vi "MSScript_SubVI_ArrayIndiceString.vi"(11 "indice string in":string) -> (1 "x:y":i32[](array[numeric]), 2 "Indice string?":bool, 3 "Array indice string out":string)   [LabVIEW 2018, in "MSScript.lvclass"]
uses:
  MSScript.lvclass
  MSScript_Transform_UInt.vi
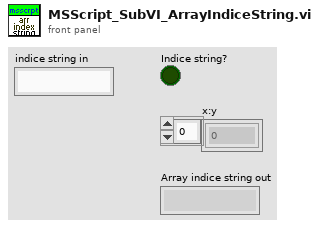
[diagram p1: front panel]
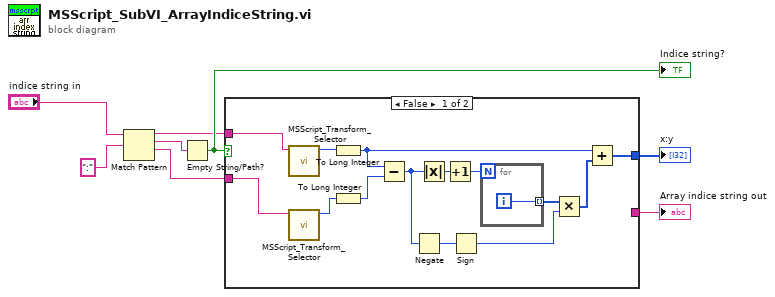
[diagram p0: block diagram]
diagram:
  n1 = Match Pattern(string="indice string in", regular expression=":") -> (before substring=w3:string, match substring=w2:string, after substring=w4:string)  [unwired: 1 in, 1 out]
  n2 = Empty String/Path?(string/path=w2) -> (empty?=w6:bool)
  "Indice string?" <- w6
  n3 = case shown="False" w6 {
    tunnel: w3 -> [w18 w24]
    tunnel: w4 -> [w16 _]
    tunnel: [w19 _] -> w5
    tunnel: [_ w24] -> w8
    frame False {
      n4 = call-poly "MSScript_Transform_Selector.vi"("string in"=w18) -> ("Value Output"=w17:u64)  [unwired: 8 in, 2 out]
      n5 = call-poly "MSScript_Transform_Selector.vi"("string in"=w16) -> ("Value Output"=w15:u64)  [unwired: 8 in, 2 out]
      n6 = To Long Integer(number=w17) -> (32bit integer=w20:i32)
      n7 = To Long Integer(number=w15) -> (32bit integer=w22:i32)
      n8 = Subtract(x=w20, y=w22) -> (x-y=w14:i32)
      n9 = Negate(x=w14) -> (-x=w11:i32)
      n10 = Absolute Value(x=w14) -> (abs(x)=w13:i32)
      n11 = Increment(x=w13) -> (x+1=w12:i32)
      n12 = Sign(1:w11) -> (0:w9:i32)
      n13 = for {
        N: w12 -> [_]
        tunnel: [w23] -> w21 mode=indexing
        i -> [w23]
      }
      n14 = Multiply(x=w21, y=w9) -> (x*y=w10:i32[])
      n15 = Add(x=w20, y=w10) -> (x+y=w19:i32[])
    }
    frame True {
    }
  }
  "x:y" <- w5
  "Array indice string out" <- w8
